vi "TEk_acquis_new.vi"() -> ()   [LabVIEW 2022 SP3]
uses:
  <vilib>/Analysis/2dsp.llb/Real FFT.vi
  <instrlib>/Tektronix TDS 200 1000 2000 Series/Tektronix TDS 200 1000 2000 Series.lvlib
  <vilib>/measure/NI_MABase.lvlib
  <vilib>/Analysis/NI_AALPro.lvlib
panel:
  out "mean of median of in phase":dbl
  out "Median in phase voltage":dbl[](array[numeric])
  out "In phase array w/ subset deleted":dbl[](array[numeric])
  out "size(s)":i32
  in  "sampling info":cluster{"Fs":dbl, "#s":dbl}={"Fs"=1000.0, "#s"=1000.0} {"Fs" format="%.2p"}
  in  "frequency of \nreference wave":dbl=10.0 format="%0.2p"
  out "0 deg vol":dbl
  out "90 deg vol":dbl
  out "Cosine reference":dbl[](graph)
  out "Sine Reference":dbl[](graph)
  out "sqrt(V1^2+V2^2)":dbl
  out "arctan(x)":dbl
  out "size(s)":i32
  out "Quadrature array w/ subset deleted":dbl[](array[numeric])
  out "Median Quadrature voltage":dbl[](array[numeric])
  out "mean of median of quadrature":dbl
  in  "Source (0: Channel 1)":u16(ring) items=["Channel 1", "Channel 2", "Channel 3", "Channel 4", "Math", "Reference A", "Reference B", "Reference C", "Reference D"]
  in  "Serial Configuration":T1={"Baud Rate"=9600, "Parity"=0, "Stop Bits"=10, "Flow Control"=2} {"Flow Control" items=["None", "XON/XOFF", "RTS/CTS", "XON/XOFF & RTS/CTS", "DTR/DSR", "XON/XOFF & DTR/DSR"]; "Stop Bits" items=["1.0"=10, "1.5"=15, "2.0"=20]; "Parity" items=["None", "Odd", "Even", "Mark", "Space"]; "Baud Rate" items=["300"=300, "600"=600, "1200"=1200, "2400"=2400, "4800"=4800, "9600"=9600, "19200"=19200]}
  out "Waveform Data":waveform(dbl)(graph)
  in  "stop":bool
  in  "Probe Attenuation (0.1)":dbl=10.0
  in  "Timeout (10000 ms)":u32=10000
  in  "VISA resource name":refnum<visa-resource-name>
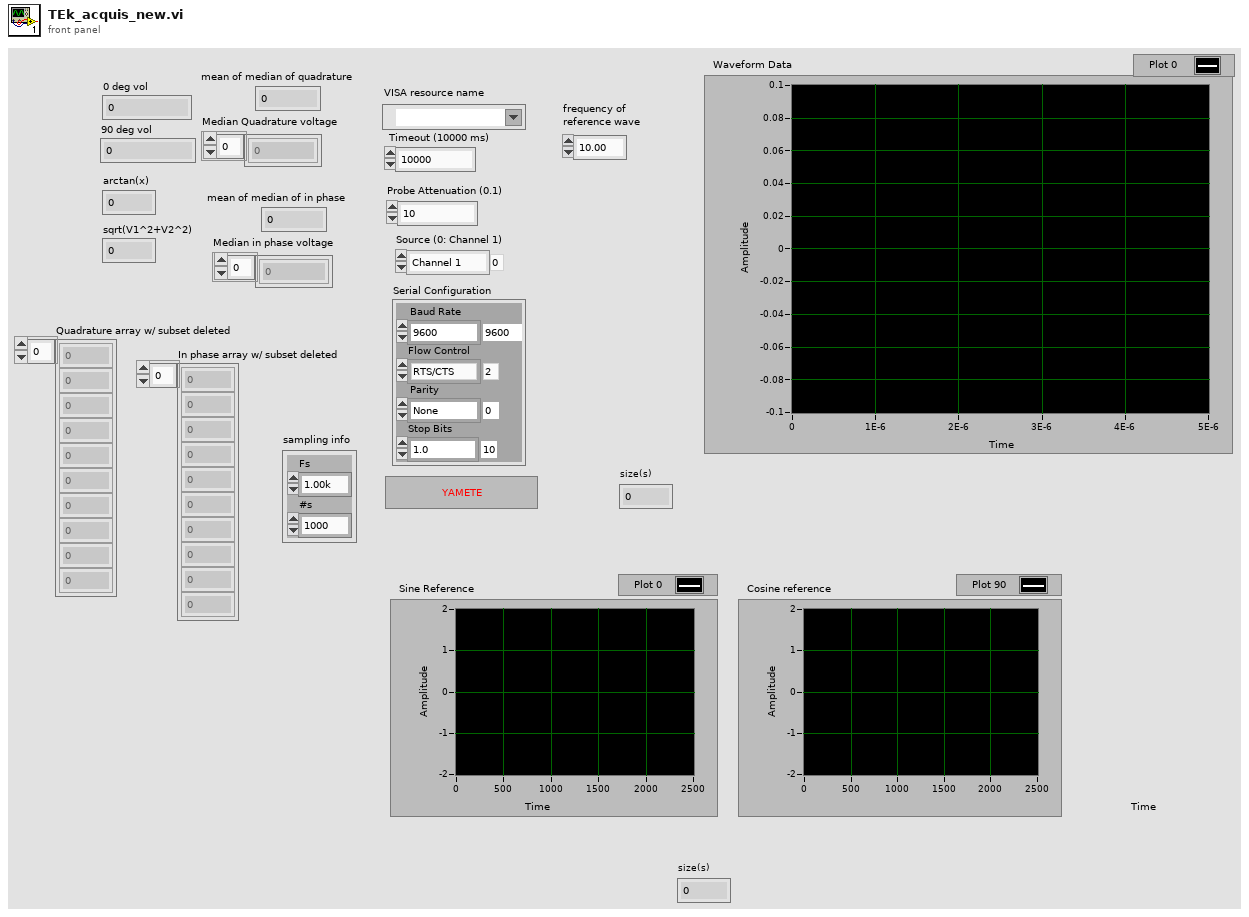
[diagram p1: front panel]
types:
  T1 = cluster{"Baud Rate":u32, "Parity":u16, "Stop Bits":u16, "Flow Control":u16}
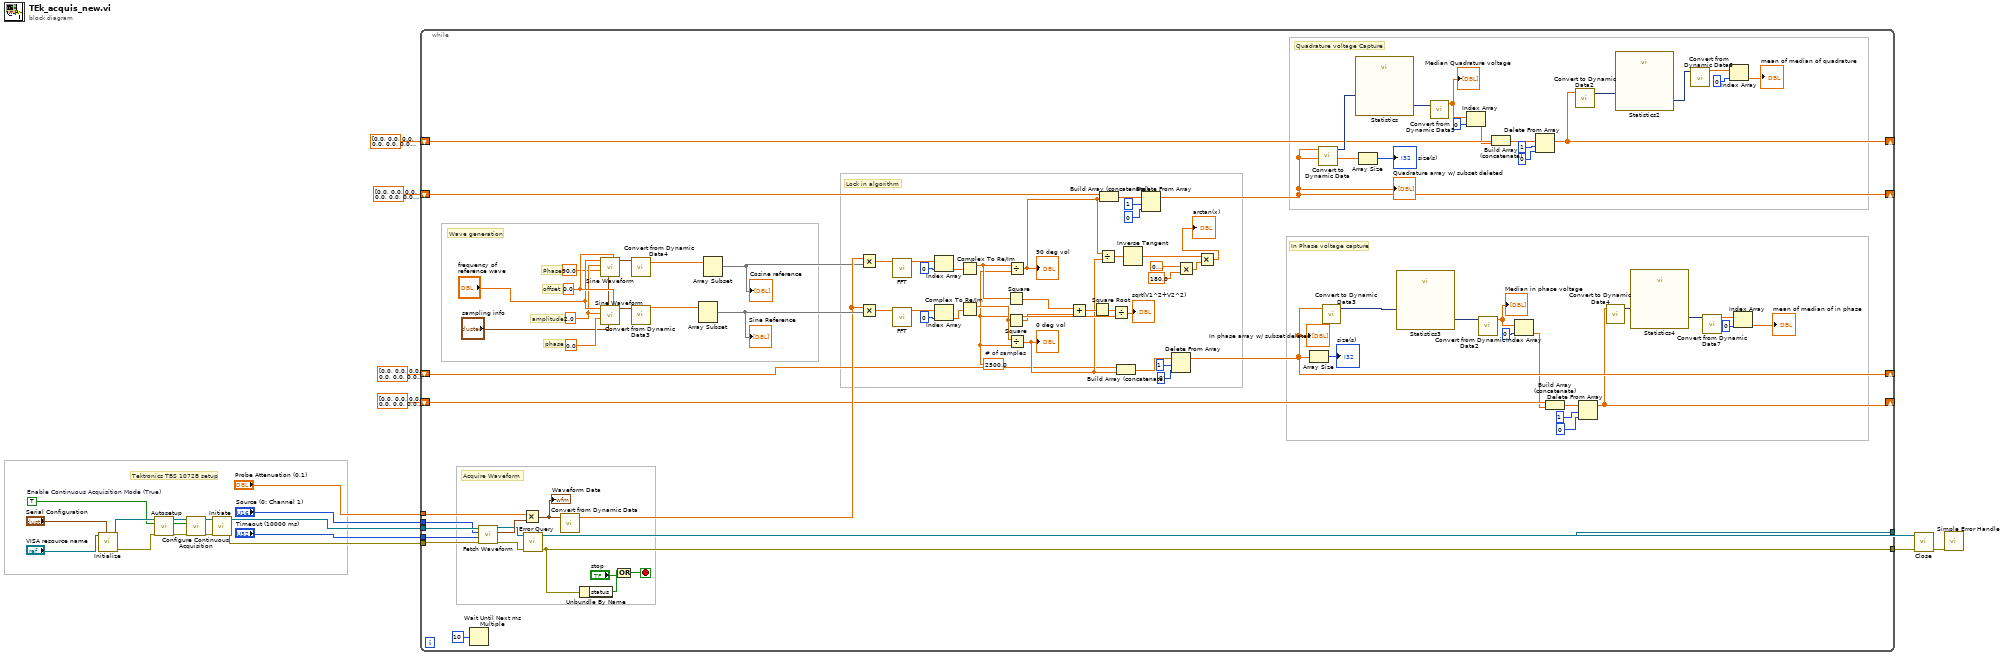
[diagram p0: block diagram]
diagram:
  w14 = TRUE  # Enable Continuous Acquisition Mode (True)
  # "Tektronics TBS 1072B setup"
  n1 = call <instrlib>:"Initialize.vi"("Serial Configuration"="Serial Configuration", "VISA resource name"="VISA resource name") -> ("error out"=w19:errorcluster, "VISA resource name out"=w18:refnum<visa-resource-name>)  [unwired: 3 in, 5 out]
  n2 = call <instrlib>:"Autosetup.vi"("error in (no error)"=w19, "VISA resource name"=w18) -> ("error out"=w16:errorcluster, "VISA resource name out"=w15:refnum<visa-resource-name>)  [unwired: 8 out]
  n3 = call <instrlib>:"Configure Continuous Acquisition.vi"("error in (no error)"=w16, "Enable Continuous Acquisition Mode (True)"=w14, "VISA resource name"=w15) -> ("error out"=w13:errorcluster, "VISA resource name out"=w12:refnum<visa-resource-name>)  [unwired: 7 out]
  n4 = call <instrlib>:"Initiate.vi"("error in (no error)"=w13, "VISA resource name"=w12) -> ("error out"=w10:errorcluster, "VISA resource name out"=w11:refnum<visa-resource-name>)  [unwired: 8 out]
  n5 = while {
    shift-right: [w79] -> _
    shift-left: dbl[] [0.0, 0.0, 0.0, 0.0, 0.0, 0.0, 0.0, 0.0, 0.0, 0.0, 0.0] -> [w84]
    shift-right: [w69] -> _
    shift-left: dbl[] [0.0, 0.0, 0.0, 0.0, 0.0, 0.0, 0.0, 0.0, 0.0, 0.0, 0.0] -> [w71]
    tunnel: w11 -> [w63]
    tunnel: w10 -> [w62]
    tunnel: "Timeout (10000 ms)" -> [w61]
    tunnel: "Probe Attenuation (0.1)" -> [w60]
    tunnel: "Source (0: Channel 1)" -> [w59]
    tunnel: [w58] -> w6
    tunnel: [w57] -> w5
    shift-right: [w36] -> _
    shift-left: dbl[] [0.0, 0.0, 0.0, 0.0, 0.0, 0.0, 0.0, 0.0, 0.0, 0.0, 0.0] -> [w41]
    shift-right: [w29] -> _
    shift-left: dbl[] [0.0, 0.0, 0.0, 0.0, 0.0, 0.0, 0.0, 0.0, 0.0, 0.0, 0.0] -> [w28]
    stop <- w50 stop-if-true
    w48 = 2500.0  # # of samples
    w115 = 0.0 ("offset")
    w113 = 2.0 ("amplitude")
    # "In Phase voltage capture"
    # "Quadrature voltage Capture"
    # "Lock in algorithm"
    # "Wave generation"
    # "amplitude"
    # "phase"
    # "offset"
    # "Phase"
    # "Acquire Waveform"
    n6 = Wait Until Next ms Multiple(millisecond multiple=u32 10) -> ()  [unwired: 1 out]
    n7 = call <instrlib>:"Fetch Waveform.vi"("error in (no error)"=w62, "Timeout (10000 ms)"=w61, "Source (0: Channel 1)"=w59, "VISA resource name"=w63) -> ("error out"=w52:errorcluster, "Waveform Data"=w56:waveform(dbl), "VISA resource name out"=w51:refnum<visa-resource-name>)  [unwired: 5 out]
    n8 = Multiply(x=w60, y=w56) -> (x*y=w47:waveform(dbl))
    "Waveform Data" <- w47
    n9 = call <instrlib>:"Error Query.vi"("error in (no error)"=w52, "VISA resource name"=w51) -> ("error out"=w57:errorcluster, "VISA resource name out"=w58:refnum<visa-resource-name>)  [unwired: 8 out]
    n10 = call "Convert from Dynamic Data"("Dynamic Data Type"=w47) -> ("Array"=w49:dbl[])  [unwired: 3 in]
    n11 = Unbundle By Name(w57) -> ("status"=w54:bool)
    n12 = call <vilib>:"Sine Waveform.vi"("offset"=w115, "sampling info"="sampling info", "phase"=90.0, "amplitude"=w113, "frequency"="frequency of \nreference wave") -> ("signal out"=w100:waveform(dbl))  [unwired: 5 in, 1 out]
    n13 = call <vilib>:"Sine Waveform.vi"("offset"=w115, "sampling info"="sampling info", "phase"=0.0, "amplitude"=w113, "frequency"="frequency of \nreference wave") -> ("signal out"=w101:waveform(dbl))  [unwired: 5 in, 1 out]
    n14 = Or(x=w54, y="stop") -> (x .or. y?=w50:bool)
    n15 = call "Convert from Dynamic Data4"("Dynamic Data Type"=w100) -> ("Array"=w94:dbl[])  [unwired: 3 in]
    n16 = call "Convert from Dynamic Data3"("Dynamic Data Type"=w101) -> ("Array"=w87:dbl[])  [unwired: 3 in]
    n17 = Array Subset(array=w87) -> (w95:dbl[])  [unwired: 2 in]
    "Sine Reference" <- w95
    n18 = Array Subset(array=w94) -> (w25:dbl[])  [unwired: 2 in]
    "Cosine reference" <- w25
    n19 = Multiply(x=w49, y=w25) -> (x*y=w103:dbl[])
    n20 = Multiply(x=w49, y=w95) -> (x*y=w86:dbl[])
    n21 = call-poly <vilib>:"FFT.vi"("X"=w103) -> ("FFT {X}"=w104:cdb[])  [unwired: 9 in, 1 out]
    n22 = call-poly <vilib>:"FFT.vi"("X"=w86) -> ("FFT {X}"=w105:cdb[])  [unwired: 9 in, 1 out]
    n23 = Index Array(array=w104, index=0) -> (element=w106:cdb)
    n24 = Index Array(array=w105, index=0) -> (element=w107:cdb)
    n25 = Complex To Re/Im(x + iy=w106) -> (x=w98:dbl)  [unwired: 1 out]
    n26 = Complex To Re/Im(x + iy=w107) -> (x=w99:dbl)  [unwired: 1 out]
    n27 = Square(x=w98) -> (x^2=w24:dbl)
    n28 = Square(x=w99) -> (x^2=w23:dbl)
    n29 = Divide(x=w98, y=w48) -> (x/y=w85:dbl)
    "90 deg vol" <- w85
    n30 = Divide(x=w99, y=w48) -> (x/y=w42:dbl)
    "0 deg vol" <- w42
    n31 = Add(x=w24, y=w23) -> (x+y=w102:dbl)
    n32 = Square Root(x=w102) -> (sqrt(x)=w97:dbl)
    n33 = Divide(x=w85, y=w42) -> (x/y=w93:dbl)
    n34 = Build Array (concatenate)(w84, w85) -> (w81:dbl[])
    n35 = Divide(x=w97, y=w48) -> (x/y=→"sqrt(V1^2+V2^2)":dbl)
    n36 = Build Array (concatenate)(w41, w42) -> (w44:dbl[])
    n37 = Inverse Tangent(1:w93) -> (0:w92:dbl)
    n38 = Delete From Array(array=w81, length=1, index=0) -> (array with subset deleted=w79:dbl[])  [unwired: 1 out]
    "Quadrature array w/ subset deleted" <- w79
    n39 = Delete From Array(array=w44, length=1, index=0) -> (array with subset deleted=w36:dbl[])  [unwired: 1 out]
    "In phase array w/ subset deleted" <- w36
    n40 = Multiply(x=0.3183098861837907, y=180.0) -> (x*y=w89:dbl)
    n41 = Multiply(x=w92, y=w89) -> (x*y=→"arctan(x)":dbl)
    n42 = Array Size(array=w36) -> (size(s)=→"size(s)":i32)
    n43 = call "Convert to Dynamic Data"("Array"=w79) -> ("Dynamic Data Type"=w78:dynamicdata)  [unwired: 3 in]
    n44 = call "Convert to Dynamic Data3"("Array"=w36) -> ("Dynamic Data Type"=w40:dynamicdata)  [unwired: 3 in]
    n45 = call "Statistics"("Signals"=w78) -> ("Median"=w77:dynamicdata)  [unwired: 25 in, 1 out]
    n46 = Array Size(array=w79) -> (size(s)=→"size(s)":i32)
    n47 = call "Statistics3"("Signals"=w40) -> ("Median"=w39:dynamicdata)  [unwired: 25 in, 1 out]
    n48 = call "Convert from Dynamic Data5"("Dynamic Data Type"=w77) -> ("Array"=w73:dbl[])  [unwired: 3 in]
    "Median Quadrature voltage" <- w73
    n49 = Index Array(array=w73, index=0) -> (element=w70:dbl)
    n50 = call "Convert from Dynamic Data2"("Dynamic Data Type"=w39) -> ("Array"=w38:dbl[])  [unwired: 3 in]
    "Median in phase voltage" <- w38
    n51 = Build Array (concatenate)(w71, w70) -> (w74:dbl[])
    n52 = Index Array(array=w38, index=0) -> (element=w27:dbl)
    n53 = Delete From Array(array=w74, length=1, index=0) -> (array with subset deleted=w69:dbl[])  [unwired: 1 out]
    n54 = Build Array (concatenate)(w28, w27) -> (w33:dbl[])
    n55 = call "Convert to Dynamic Data2"("Array"=w69) -> ("Dynamic Data Type"=w68:dynamicdata)  [unwired: 3 in]
    n56 = Delete From Array(array=w33, length=1, index=0) -> (array with subset deleted=w29:dbl[])  [unwired: 1 out]
    n57 = call "Convert to Dynamic Data4"("Array"=w29) -> ("Dynamic Data Type"=w30:dynamicdata)  [unwired: 3 in]
    n58 = call "Statistics2"("Signals"=w68) -> ("Arithmetic Mean"=w67:dynamicdata)  [unwired: 25 in, 1 out]
    n59 = call "Statistics4"("Signals"=w30) -> ("Arithmetic Mean"=w26:dynamicdata)  [unwired: 25 in, 1 out]
    n60 = call "Convert from Dynamic Data6"("Dynamic Data Type"=w67) -> ("Array"=w66:dbl[])  [unwired: 3 in]
    n61 = call "Convert from Dynamic Data7"("Dynamic Data Type"=w26) -> ("Array"=w32:dbl[])  [unwired: 3 in]
    n62 = Index Array(array=w66, index=0) -> (element=→"mean of median of quadrature":dbl)
    n63 = Index Array(array=w32, index=0) -> (element=→"mean of median of in phase":dbl)
  }
  n64 = call <instrlib>:"Close.vi"("error in (no error)"=w5, "VISA resource name"=w6) -> ("error out"=w21:errorcluster)  [unwired: 9 out]
  n65 = call <vilib>:"Simple Error Handler.vi"("error in (no error)"=w21) -> ()  [unwired: 1 in, 8 out]
